vi "8.1.SubVI 计数器.vi"(11 "布尔":bool) -> (3 "数值":u8)   [LabVIEW 2019]
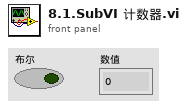
[diagram p1: front panel]
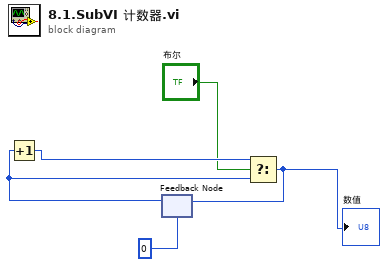
[diagram p0: block diagram]
diagram:
  n1 = feedback #1(u8 0) -> (w4:u8)
  n2 = Increment(x=w4) -> (x+1=w3:u8)
  n3 = Select(t=w3, s="布尔", f=w4) -> (s? t:f=w5:u8)
  "数值" <- w5
  n4 = feedback-in #1(w5) -> ()
